vi "J1939 Address Lookup Table.vi"(7 "Action":T2, 8 "error in (no error)":errorcluster, 10 "Address":u8, 11 "Data":T1 {"Name" format="%.0x"}) -> (0 "error out":errorcluster, 1 "All Data":T1[](array[typedef]) {"Name" format="%.0x"}, 2 "Found?":bool, 3 "Data":T1 {"Name" format="%.0x"})   [LabVIEW 2013, in "J1939.lvlib"]
uses:
  J1939.lvlib
  Internals/LUTs/J1939 Address Lookup Table Data.ctl
  Internals/LUTs/J1939 Address Lookup Table Action.ctl
panel:
  # "OUTPUTS"
  # "INPUTS"
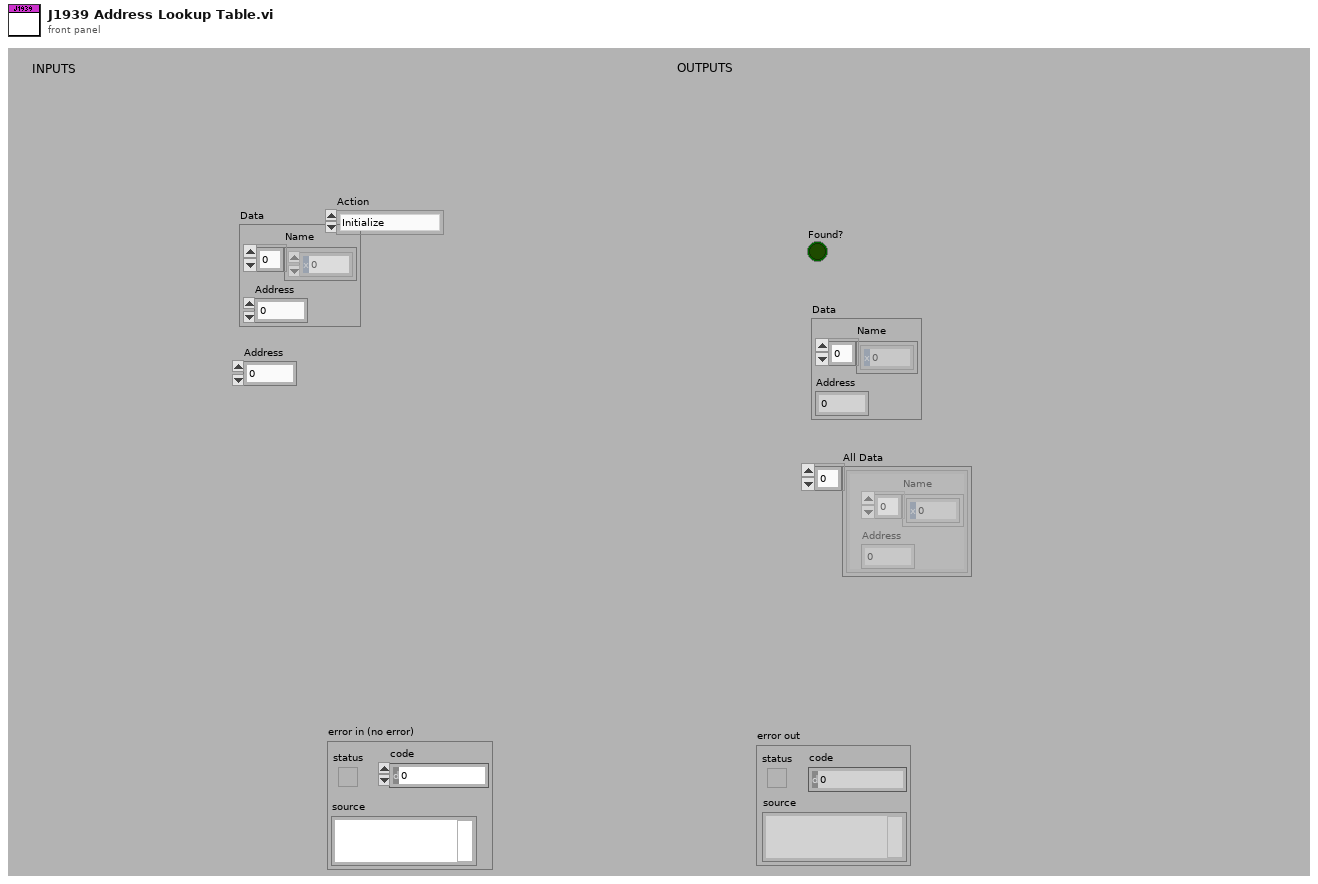
[diagram p1: front panel]
types:
  T1 = typedef "J1939.lvlib/J1939 Address Lookup Table Data.ctl" = cluster{"Name":u8[], "Address":u8}
  T2 = typedef "J1939.lvlib/J1939 Address Lookup Table Action.ctl" = enum16{"Initialize", "Add", "Get", "Remove", "Get All"}
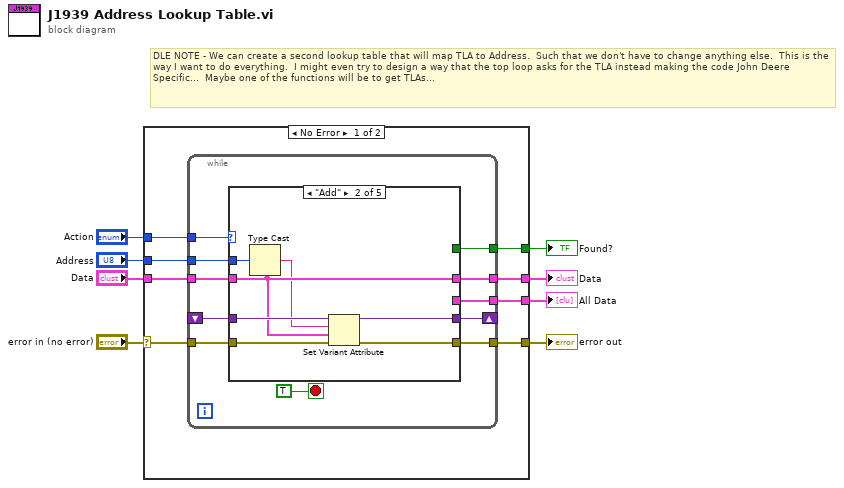
[diagram p0: block diagram]
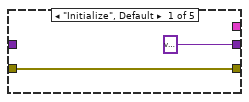
[diagram p2: hidden frame]
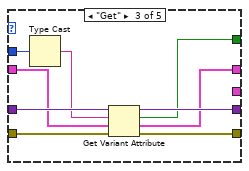
[diagram p3: hidden frame]
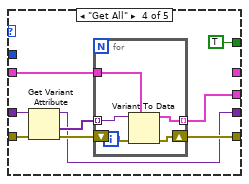
[diagram p4: hidden frame]
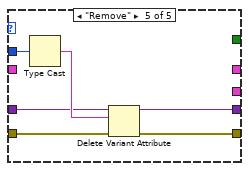
[diagram p5: hidden frame]
diagram:
  # "DLE NOTE - We can create a second lookup table that will map TLA to Address.  Such that we don't have to change anything else.  This is the way I want to do everything.  I might even try to design a way that the top loop asks for the TLA instead making the code John Deere Specific...  Maybe one of the functions will be to get TLAs..."
  n1 = case shown="No Error" "error in (no error)" {
    selector: "error in (no error)" -> [w12 w66]
    tunnel: [w11 w66] -> w7
    tunnel: "Data" -> [w15 _]
    tunnel: "Action" -> [w16 _]
    tunnel: [w14 _] -> w4
    tunnel: "Address" -> [w13 _]
    tunnel: [w10 _] -> w2
    tunnel: [w9 _] -> w1
    frame No Error {
      n2 = while {
        shift-right: [w26] -> _
        shift-left: _ -> [w25]
        tunnel: w16 -> [w27]
        tunnel: w15 -> [w18]
        tunnel: [w23] -> w14
        tunnel: w13 -> [w22]
        tunnel: w12 -> [w21]
        tunnel: [w20] -> w11
        tunnel: [w19] -> w10
        tunnel: [w17] -> w9
        stop <- TRUE stop-if-true
        n3 = case shown="\"Add\"" w27 {
          tunnel: [variant ("duplicate variant") w35 w44 w47 w60] -> w26
          tunnel: w25 -> [_ w36 w45 w54 w61]
          tunnel: [_ w34 w38 _ _] -> w23
          tunnel: w22 -> [_ w33 w43 _ w65]
          tunnel: w21 -> [w28 w31 w41 w53 w64]
          tunnel: [w28 w30 w40 w48 w63] -> w20
          tunnel: [_ _ w37 TRUE _] -> w19
          tunnel: w18 -> [_ w34 w39 w50 _]
          tunnel: [_ _ _ w46 _] -> w17
          frame "Initialize", Default {
          }
          frame "Add" {
            n4 = Type Cast(x=w33) -> (*(type *) &x=w32:string)  [unwired: 1 in]
            n5 = Set Variant Attribute(Variant=w36, name=w32, value=w34, error in=w31) -> (Variant out=w35:variant, error out=w30:errorcluster)  [unwired: 1 out]
          }
          frame "Get" {
            n6 = Type Cast(x=w43) -> (*(type *) &x=w42:string)  [unwired: 1 in]
            n7 = Get Variant Attribute(Variant=w45, name=w42, default value (empty Variant)=w39, error in=w41) -> (duplicate Variant=w44:variant, found=w37:bool, value=w38:T1, error out=w40:errorcluster)
          }
          frame "Get All" {
            n8 = Get Variant Attribute(Variant=w54, error in=w53) -> (duplicate Variant=w47:variant, values=w51:variant[], error out=w49:errorcluster)  [unwired: 2 in, 1 out]
            n9 = for {
              tunnel: w51 -> [w59] mode=indexing
              tunnel: w50 -> [w58]
              shift-right: [w56] -> w48
              shift-left: w49 -> [w57]
              tunnel: [w55] -> w46 mode=indexing
              n10 = Variant To Data(error in=w57, type=w58, Variant=w59) -> (data=w55:T1, error out=w56:errorcluster)
            }
          }
          frame "Remove" {
            n11 = Type Cast(x=w65) -> (*(type *) &x=w62:string)  [unwired: 1 in]
            n12 = Delete Variant Attribute(4:w64, 6:w62, 7:w61) -> (0:w63:errorcluster, 3:w60:variant)  [unwired: 1 out]
          }
        }
      }
    }
    frame Error {
    }
  }
  "error out" <- w7
  "Data" <- w4
  "Found?" <- w2
  "All Data" <- w1
